vi "start.vi"(8 "error in (no error)":errorcluster, 11 "FlowControlValveCompensator in":refnum<class "FlowControlValveCompensator.lvclass">) -> (0 "error out":errorcluster, 3 "FlowControlValveCompensator out":refnum<class "FlowControlValveCompensator.lvclass">)   [LabVIEW 2013, in "FlowControlValveCompensator.lvclass"]
uses:
  FlowControlValveCompensator.lvclass
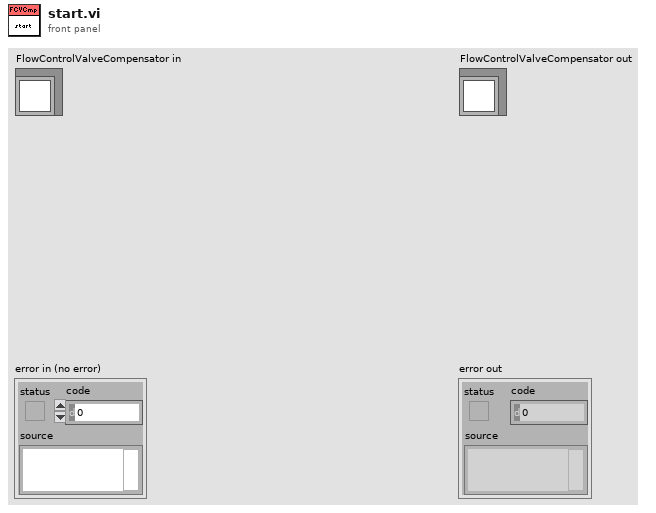
[diagram p1: front panel]
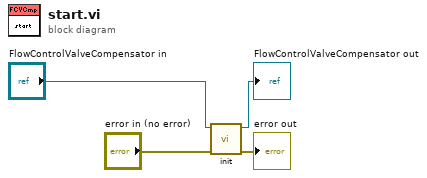
[diagram p0: block diagram]
diagram:
  n1 = call-dynamic "init.vi"("error in (no error)"="error in (no error)", "FlowControlValveCompensator in"="FlowControlValveCompensator in") -> ("error out"=→"error out":errorcluster, "FlowControlValveCompensator out"=→"FlowControlValveCompensator out":refnum<class "FlowControlValveCompensator.lvclass">)  [unwired: 8 in]
